vi "Send Stop.vi"(8 "error in":errorcluster, 11 "GUI in":refnum<class "GUI.lvclass">) -> (0 "error out":errorcluster, 3 "GUI out":refnum<class "GUI.lvclass">)   [LabVIEW 2015, in "GUI.lvclass"]
doc: "Send the stop command to every GUI registered with the facade. The GUIs themselves will be responsible for handling the stop notifier (i.e. destroying the reference)."
uses:
  GUI.lvclass
  GUI.lvclass/GUI.ctl
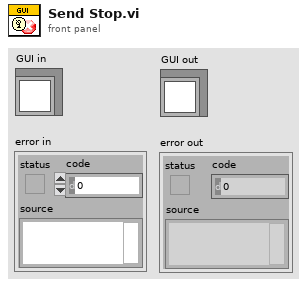
[diagram p1: front panel]
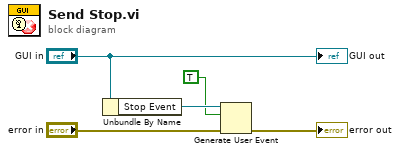
[diagram p0: block diagram]
diagram:
  n1 = Unbundle By Name("GUI in") -> ("Stop Event"=w2:refnum<user-event>)
  n2 = Generate User Event(user event=w2, event data cluster=TRUE ("event data"), error in="error in") -> (error out=→"error out":errorcluster)  [unwired: 1 in, 1 out]
  "GUI out" <- "GUI in"
